vi "pco.camera_LightSheet_Example_IMAQ.vi"() -> ()   [LabVIEW 2019]
uses:
  pco.camera/Camera.lvclass
  pco.sdk/SpecialCommandsEdge/SpecialCommandsEdge.lvlib
panel:
  in  "dwExposureLines":u32=100
  in  "wTimeBase":u16(ring)=1 items=["ns", "us", "ms"]
  in  "dwLineTime":u32=50
  out "rawImage":u16[][](array[numeric])
  out "Image":T1(plugin-control)
  in  "data_format":T2(ring)=enum."Mono16"
  in  "Image Index":u32 max=99
  out "Recorded Images":u32
  in  "Quit":bool
  in  "roiY1":u64=2 min=2 max=1040 step=1
  in  "roiX1":u64=2 min=2 max=1392 step=1
  in  "roiY0":u64=1 min=1 max=1039 step=1
  in  "roiX0":u64=1 min=1 max=1391 step=1
  out "Image Height":u64
  out "Image Width":u64
  in  "dwImgCount":u32=10 caption="Required Number of Images" max=4023
  out "Error":errorcluster {"code" format="%x"}
  # "This example is similar to the simple example, but uses get/set line timeing for controlling the exposure.\nExposureTime = LineTime * ExposureLines\nBeside of the line timing part, a simple recording of an image sequence and the image access afterwards is done.\nIt is a good starting point for writing own applications, especially  for light sheet application development.\nBut it will not be fail save, i.e. doesnt react on errors, just handles them forward to the end\n\nUsage:\nSelect your required image count and the required line tiime + number of exposure lines before you start the program.\nOnce started, the camera class will be initialized and images will be recorded automatically.\nWhen acquisition has finished you can address the images and set a certain roi \nTo finish the program click on quit application, this will force fan exit of the camera class"
  # "pco.labview"
  # "Camera Setup"
  # "Recording Control"
  # "Parameters for image readout"
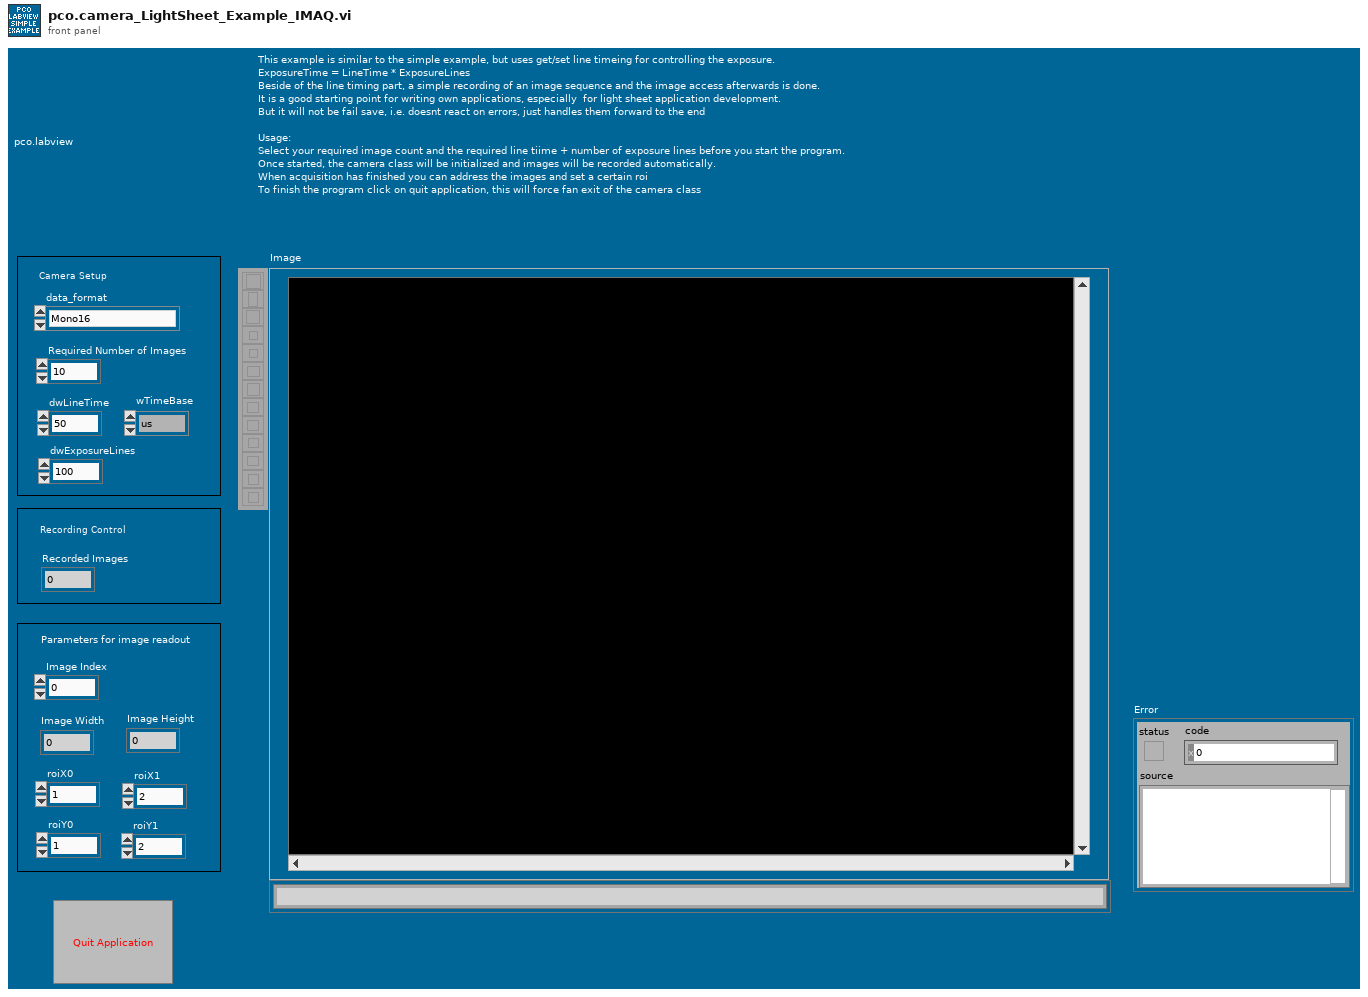
[diagram p1: front panel]
types:
  T1 = typedef "IMAQ Image.ctl" = refnum<image>
  T2 = enum16{"Undefined", "Mono8", "Mono16", "BGRA8", "RGBA8", "BGRA16", "RGBA16", "CompressedMono8"}
  T3 = enum8{"Enabled", "Disabled", "Disabled and Grayed Out"}
  T4 = enum16{"sequence", "sequence non blocking", "ring buffer", "fifo", "sequence_dpcore", "sequence_non_blocking_dpcore", "ring_buffer_dpcore", "fifo_dpcore", "tif", "multitif", "pcoraw", "b16", "dicom", "multidicom"}
  T5 = typedef "Image Type" = u32
  T6 = typedef "Camera.lvclass/binning.ctl" = cluster{"vert":u16, "horz":u16}
  T7 = cluster{"exposure_time_s":dbl, "delay_time_s":dbl, "roi":cluster{"x0":u64, "y0":u64, "x1":u64, "y1":u64}, "timestamp_mode":u16, "pixelrate":u32, "trigger_mode":u16, "acquire_mode":u16, "metadata_mode":u16, "noisefilter_mode":u16, "binning":T6}
  T8 = typedef "Color (U64)" = cluster{"Plane 3 (Blue)":u16, "Plane 2 (Green)":u16, "Plane 1 (Red)":u16, "Plane 4 (alpha)":u16}
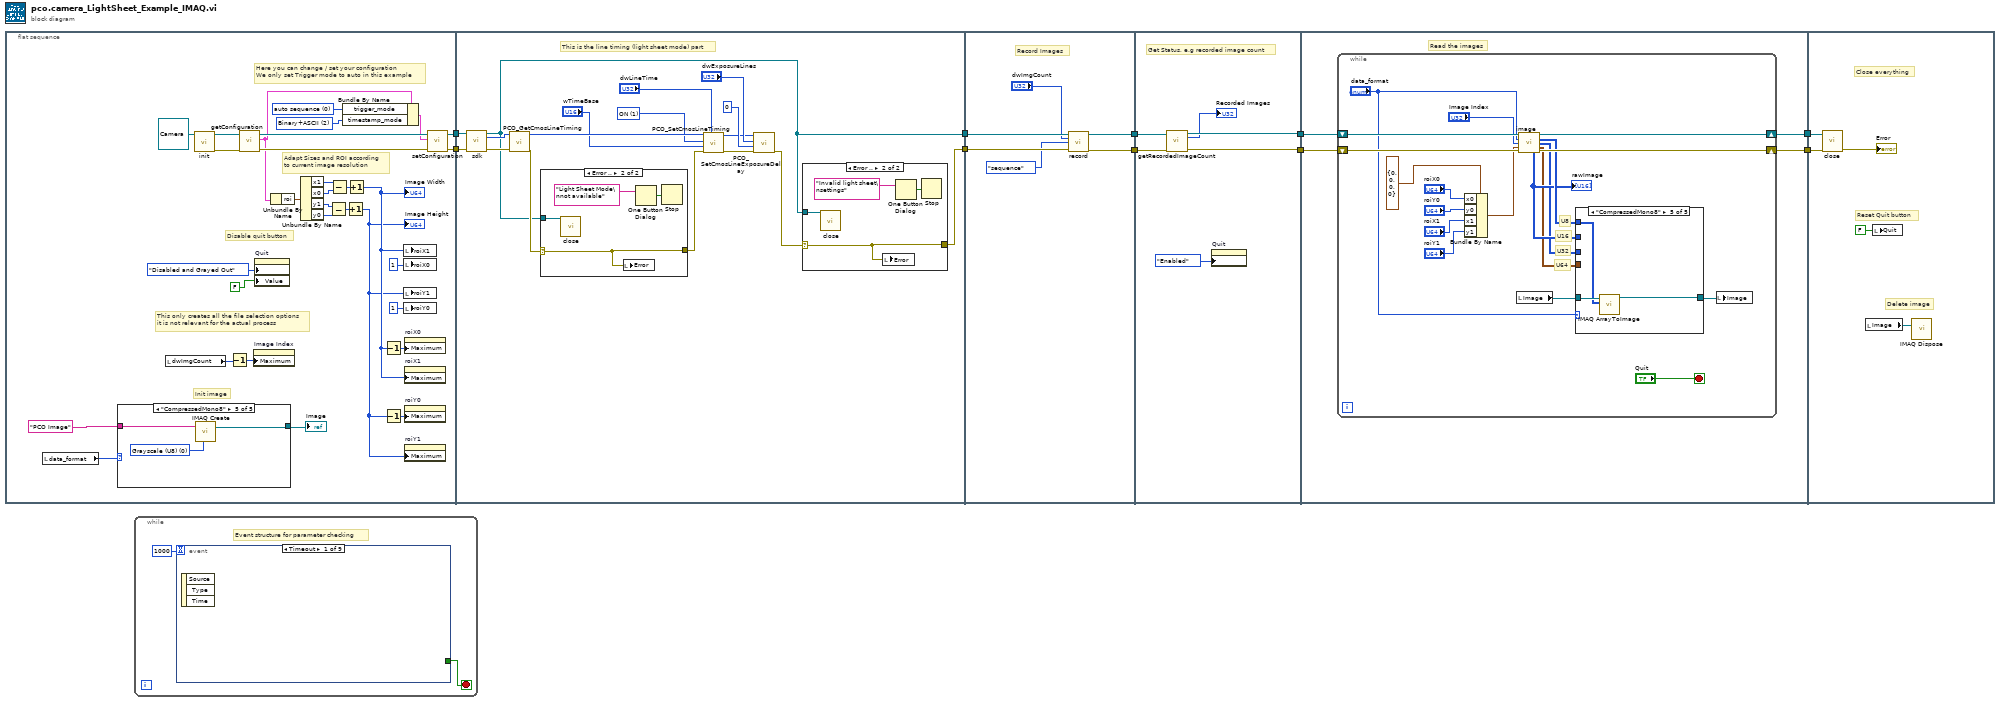
[diagram p0: block diagram]
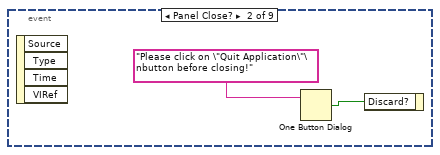
[diagram p2: hidden frame]
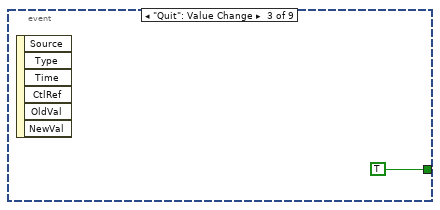
[diagram p3: hidden frame]
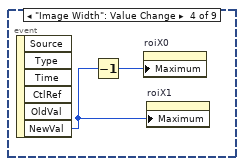
[diagram p4: hidden frame]
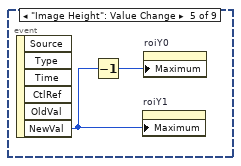
[diagram p5: hidden frame]
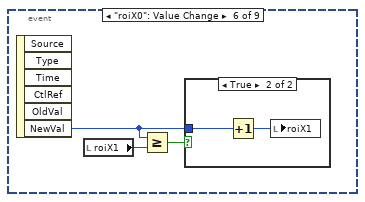
[diagram p6: hidden frame]
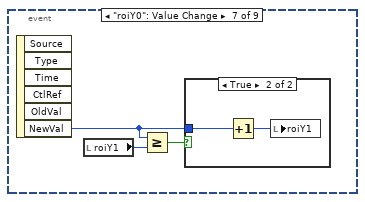
[diagram p8: hidden frame]
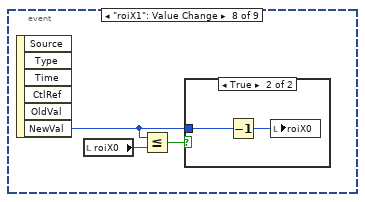
[diagram p10: hidden frame]
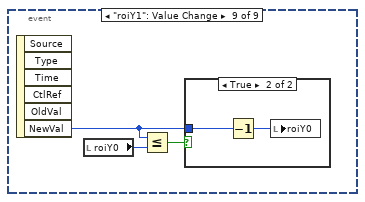
[diagram p12: hidden frame]
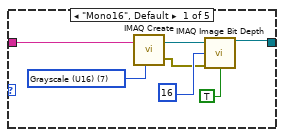
[diagram p14: hidden frame]
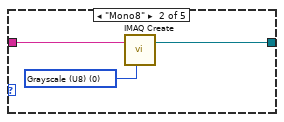
[diagram p15: hidden frame]
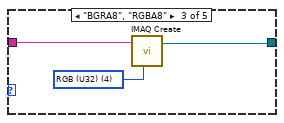
[diagram p16: hidden frame]
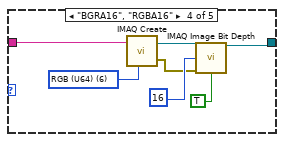
[diagram p17: hidden frame]
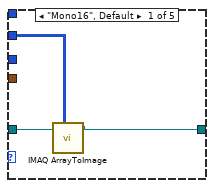
[diagram p20: hidden frame]
diagram:
  n1 = flat-sequence {
    tunnel: [w34] -> w4
    tunnel: [w33] -> w2
    tunnel: w4 -> [w77]
    tunnel: [w65] -> w3
    tunnel: w2 -> [w76]
    tunnel: [w66] -> w1
    tunnel: w3 -> [w97]
    tunnel: w1 -> [w96]
    tunnel: [w94] -> w10
    tunnel: [w93] -> w9
    tunnel: w10 -> [w103]
    tunnel: w9 -> [w102]
    tunnel: [w101] -> w8
    tunnel: [w100] -> w7
    tunnel: w8 -> [w106]
    tunnel: w7 -> [w107]
    tunnel: [w105] -> w6
    tunnel: [w104] -> w5
    tunnel: w6 -> [w144]
    tunnel: w5 -> [w143]
    frame #0 {
      w18 = u16 2 items=["OFF", "Binary", "Binary+ASCII", "ASCII"] ("TimestampMode")
      w38 = u16 0 items=["auto sequence"=0, "software trigger"=1, "external exposure start & software trigger"=2, "external exposure control"=3, "external synchronized"=4, "fast external exposure control"=5, "external CDS control"=6, "slow external exposure control"=7, "external synchronized HDSDI"=258] ("TriggerMode")
      # "Init image"
      # "This only creates all the file selection options\nit is not relevant for the actual process"
      # "Adapt Sizes and ROI according\nto current image resolution"
      # "Disable quit button"
      # "Here you can change / set your configuration\nWe only set Trigger mode to auto in this example"
      n2 = local read "data_format"() -> (w13:T2)
      n3 = case shown="\"CompressedMono8\"" w13 {
        tunnel: "PCO Image" ("Image Name") -> [w47 w51 w53 w60 w63]
        tunnel: [w42 w49 w52 w56 w62] -> w12
        frame "Mono16", Default {
          w48 = T5 7 items=["Grayscale (U8)", "Grayscale (I16)", "Grayscale (SGL)", "Complex (CSG)", "RGB (U32)", "HSL (U32)", "RGB (U64)", "Grayscale (U16)"] ("Image Type")
          n4 = call "IMAQ Create"("Image Name"=w47, "Image Type"=w48) -> ("New Image"=w44:T1, "error out"=w43:errorcluster)  [unwired: 3 in]
          n5 = call "IMAQ Image Bit Depth"("Image"=w44, "Bit Depth (0)"=u32 16, "error in (no error)"=w43, "Get/Set Bit Depth? (Set)"=TRUE) -> ("Image Out"=w42:T1)  [unwired: 9 in, 2 out]
        }
        frame "Mono8" {
          w50 = T5 0 items=["Grayscale (U8)", "Grayscale (I16)", "Grayscale (SGL)", "Complex (CSG)", "RGB (U32)", "HSL (U32)", "RGB (U64)", "Grayscale (U16)"] ("Image Type")
          n6 = call "IMAQ Create"("Image Name"=w51, "Image Type"=w50) -> ("New Image"=w49:T1)  [unwired: 3 in, 1 out]
        }
        frame "BGRA8", "RGBA8" {
          w54 = T5 4 items=["Grayscale (U8)", "Grayscale (I16)", "Grayscale (SGL)", "Complex (CSG)", "RGB (U32)", "HSL (U32)", "RGB (U64)", "Grayscale (U16)"] ("Image Type")
          n7 = call "IMAQ Create"("Image Name"=w53, "Image Type"=w54) -> ("New Image"=w52:T1)  [unwired: 3 in, 1 out]
        }
        frame "BGRA16", "RGBA16" {
          w61 = T5 6 items=["Grayscale (U8)", "Grayscale (I16)", "Grayscale (SGL)", "Complex (CSG)", "RGB (U32)", "HSL (U32)", "RGB (U64)", "Grayscale (U16)"] ("Image Type")
          n8 = call "IMAQ Create"("Image Name"=w60, "Image Type"=w61) -> ("New Image"=w57:T1, "error out"=w55:errorcluster)  [unwired: 3 in]
          n9 = call "IMAQ Image Bit Depth"("Image"=w57, "Bit Depth (0)"=u32 16, "error in (no error)"=w55, "Get/Set Bit Depth? (Set)"=TRUE) -> ("Image Out"=w56:T1)  [unwired: 9 in, 2 out]
        }
        frame "CompressedMono8" {
          w64 = T5 0 items=["Grayscale (U8)", "Grayscale (I16)", "Grayscale (SGL)", "Complex (CSG)", "RGB (U32)", "HSL (U32)", "RGB (U64)", "Grayscale (U16)"] ("Image Type")
          n10 = call "IMAQ Create"("Image Name"=w63, "Image Type"=w64) -> ("New Image"=w62:T1)  [unwired: 3 in, 1 out]
        }
      }
      "Image" <- w12
      n11 = local read "dwImgCount"() -> (w14:u32)
      n12 = call-dynamic "init.vi"("Camera in"=refnum<class "Camera.lvclass"> refnum ("PCOCamera in")) -> ("Camera out"=w40:refnum<class "Camera.lvclass">, "error out"=w39:errorcluster)  [unwired: 8 in]
      n13 = Decrement(x=w14) -> (x-1=w15:u32)
      n14 = call-dynamic "getConfiguration.vi"("error in (no error)"=w39, "Camera in"=w40) -> ("error out"=w36:errorcluster, "configuration"=w28:T7, "Camera out"=w37:refnum<class "Camera.lvclass">)  [unwired: 7 in]
      n15 = property on="Image Index" class="DigNum (strict)"("Maximum"=w15) -> ()  [unwired: 2 in, 2 out]
      n16 = property on="Quit" class="Bool (strict)"("DisabledEnum"=T3."Disabled and Grayed Out" ("Disabled"), "Value"=FALSE ("Stop")) -> ()  [unwired: 2 in, 2 out]
      n17 = Unbundle By Name(w28) -> ("roi"=w27:cluster{"x0":u64, "y0":u64, "x1":u64, "y1":u64})
      n18 = Unbundle By Name(w27) -> ("x1"=w25:u64, "x0"=w26:u64, "y1"=w23:u64, "y0"=w24:u64)
      n19 = Subtract(x=w23, y=w24) -> (x-y=w21:u64)
      n20 = Subtract(x=w25, y=w26) -> (x-y=w22:u64)
      n21 = Bundle By Name(cluster=w28, "trigger_mode"=w38, "timestamp_mode"=w18) -> (w35:T7)
      n22 = Increment(x=w21) -> (x+1=w19:u64)
      "Image Height" <- w19
      n23 = Increment(x=w22) -> (x+1=w20:u64)
      "Image Width" <- w20
      n24 = Decrement(x=w20) -> (x-1=w30:u64)
      n25 = Decrement(x=w19) -> (x-1=w29:u64)
      n26 = local write "roiX1"(w20) -> ()
      n27 = local write "roiX0"(u64 1 ("roiY0")) -> ()
      n28 = local write "roiY1"(w19) -> ()
      n29 = local write "roiY0"(u64 1 ("roiY0")) -> ()
      n30 = property on="roiX0" class="DigNum (strict)"("Maximum"=w30) -> ()  [unwired: 2 in, 2 out]
      n31 = property on="roiX1" class="DigNum (strict)"("Maximum"=w20) -> ()  [unwired: 2 in, 2 out]
      n32 = property on="roiY0" class="DigNum (strict)"("Maximum"=w29) -> ()  [unwired: 2 in, 2 out]
      n33 = property on="roiY1" class="DigNum (strict)"("Maximum"=w19) -> ()  [unwired: 2 in, 2 out]
      n34 = call-dynamic "setConfiguration.vi"("error in (no error)"=w36, "configuration"=w35, "Camera in"=w37) -> ("error out"=w33:errorcluster, "Camera out"=w34:refnum<class "Camera.lvclass">)  [unwired: 7 in]
    }
    frame #1 {
      w73 = u16 1 items=["OFF", "ON"] ("wParameter")
      # "This is the line timing (light sheet mode) part"
      n35 = call-dynamic "sdk.vi"("Camera in"=w77, "error in (no error)"=w76) -> ("Camera out"=w65:refnum<class "Camera.lvclass">, "sdk"=w75:u64, "error out"=w81:errorcluster)  [unwired: 11 in]
      n36 = call "PCO_GetCmosLineTiming.vi"("ph"=w75, "error in (no error)"=w81) -> ("ph out"=w74:u64, "error out"=w80:errorcluster)  [unwired: 10 in, 6 out]
      n37 = case shown="Error .." w80 {
        selector: w80 -> [w87 w88]
        tunnel: [w87 w88] -> w79
        tunnel: w65 -> [_ w89]
        frame No Error {
        }
        frame Error {
          n38 = call-dynamic "close.vi"("Camera in"=w89) -> ()  [unwired: 10 in, 1 out]
          n39 = local write "Error"(w88) -> ()
          n40 = One Button Dialog(message="Light Sheet Mode\nnot available") -> (true=w90:bool)  [unwired: 1 in]
          n41 = Stop(stop? (T)=w90) -> ()
        }
      }
      n42 = call "PCO_SetCmosLineTiming.vi"("dwLineTime"="dwLineTime", "error in (no error)"=w79, "wTimeBase"="wTimeBase", "wParameter"=w73, "ph"=w74) -> ("error out"=w78:errorcluster, "ph out"=w68:u64)  [unwired: 4 in, 1 out]
      n43 = call "PCO_SetCmosLineExposureDelay.vi"("error in (no error)"=w78, "dwDelayLines"=u32 0, "dwExposureLines"="dwExposureLines", "ph"=w68) -> ("error out"=w67:errorcluster)  [unwired: 5 in, 2 out]
      n44 = case shown="Error .." w67 {
        selector: w67 -> [w82 w83]
        tunnel: [w82 w83] -> w66
        tunnel: w65 -> [_ w84]
        frame No Error {
        }
        frame Error {
          n45 = call-dynamic "close.vi"("Camera in"=w84) -> ()  [unwired: 10 in, 1 out]
          n46 = local write "Error"(w83) -> ()
          n47 = One Button Dialog(message="Invalid light sheet\nsettings") -> (true=w85:bool)  [unwired: 1 in]
          n48 = Stop(stop? (T)=w85) -> ()
        }
      }
    }
    frame #2 {
      # "Record Images"
      n49 = call-dynamic "record.vi"("Camera in"=w97, "num_images"="dwImgCount", "record_mode"=T4."sequence", "error in (no error)"=w96) -> ("Camera out"=w94:refnum<class "Camera.lvclass">, "error out"=w93:errorcluster)  [unwired: 10 in]
    }
    frame #3 {
      # "Get Status, e.g recorded image count"
      n50 = call-dynamic "getRecordedImageCount.vi"("Camera in"=w103, "error in (no error)"=w102) -> ("Camera out"=w101:refnum<class "Camera.lvclass">, "recorded_image_count"=→"Recorded Images":u32, "error out"=w100:errorcluster)  [unwired: 11 in]
      n51 = property on="Quit" class="Bool (strict)"("DisabledEnum"=T3."Enabled" ("Disabled")) -> ()  [unwired: 2 in, 2 out]
    }
    frame #4 {
      # "Read the images"
      n52 = while {
        shift-right: [w124] -> w105
        shift-left: w106 -> [w126]
        shift-right: [w119] -> w104
        shift-left: w107 -> [w125]
        stop <- "Quit" stop-if-true
        # "U64"
        # "U32"
        # "U16"
        # "U8"
        n53 = Bundle By Name(cluster=cluster{"x0":u64, "y0":u64, "x1":u64, "y1":u64} {"x0"=0, "y0"=0, "x1"=0, "y1"=0} ("roi"), "x0"="roiX0", "y0"="roiY0", "x1"="roiX1", "y1"="roiY1") -> (w118:cluster{"x0":u64, "y0":u64, "x1":u64, "y1":u64})
        n54 = local read "Image"() -> (w111:T1)
        n55 = call-dynamic "image.vi"("Camera in"=w126, "data_format"="data_format", "image_index"="Image Index", "roi"=w118, "error in (no error)"=w125) -> ("Camera out"=w124:refnum<class "Camera.lvclass">, "image (U8)"=w115:u8[][], "image (U32)"=w113:u32[][], "image (U64)"=w112:T8[][], "raw_image (U16)"=w114:u16[][], "error out"=w119:errorcluster)  [unwired: 3 in, 2 out]
        "rawImage" <- w114
        n56 = case shown="\"CompressedMono8\"" "data_format" {
          tunnel: w111 -> [w129 w132 w135 w138 w141]
          tunnel: [w127 w130 w134 w136 w140] -> w110
          tunnel: w112 -> [_ _ _ w137 _]
          tunnel: w113 -> [_ _ w133 _ _]
          tunnel: w115 -> [_ w131 _ _ w139]
          tunnel: w114 -> [w128 _ _ _ _]
          frame "Mono16", Default {
            n57 = call "IMAQ ArrayToImage"("Image Pixels (U16)"=w128, "Image"=w129) -> ("Image Out"=w127:T1)  [unwired: 8 in, 1 out]
          }
          frame "Mono8" {
            n58 = call "IMAQ ArrayToImage"("Image Pixels (U8)"=w131, "Image"=w132) -> ("Image Out"=w130:T1)  [unwired: 8 in, 1 out]
          }
          frame "BGRA8", "RGBA8" {
            n59 = call "IMAQ ArrayToColorImage"("Image Pixels (U32)"=w133, "Image"=w135) -> ("Image Out"=w134:T1)  [unwired: 3 in, 1 out]
          }
          frame "BGRA16", "RGBA16" {
            n60 = call "IMAQ ArrayToColorImage"("Image"=w138, "Image Pixels (U64)"=w137) -> ("Image Out"=w136:T1)  [unwired: 3 in, 1 out]
          }
          frame "CompressedMono8" {
            n61 = call "IMAQ ArrayToImage"("Image Pixels (U8)"=w139, "Image"=w141) -> ("Image Out"=w140:T1)  [unwired: 8 in, 1 out]
          }
        }
        n62 = local write "Image"(w110) -> ()
      }
    }
    frame #5 {
      # "Delete image"
      # "Reset Quit button"
      # "Close everything"
      n63 = call-dynamic "close.vi"("error in (no error)"=w143, "Camera in"=w144) -> ("error out"=→"Error":errorcluster)  [unwired: 9 in]
      n64 = local read "Image"() -> (w142:T1)
      n65 = local write "Quit"(FALSE ("Stop")) -> ()
      n66 = call "IMAQ Dispose"("Image"=w142) -> ()  [unwired: 5 in, 1 out]
    }
  }
  n67 = while {
    stop <- w147 stop-if-true
    # "Event structure for parameter checking"
    n68 = event shown="[0] Timeout" {
      selector: _ -> [_ _ _ _ _ _ _ _ _]
      dyn-events: _ -> [_ _ _ _ _ _ _ _ _]
      timeout: 1000 -> [_ _ _ _ _ _ _ _ _]
      tunnel: [_ _ TRUE _ _ _ _ _ _] -> w147
      event Timeout {
        n69 = event-data() -> ()  [unwired: 1 in, 3 out]
      }
      event Panel Close? {
        n70 = event-data() -> ()  [unwired: 1 in, 4 out]
        n71 = One Button Dialog(message="Please click on \"Quit Application\"\nbutton before closing!") -> (true=w149:bool)  [unwired: 1 in]
        n72 = event-data("Discard?"=w149) -> ()  [unwired: 1 in, 1 out]
      }
      event "Quit": Value Change {
        n73 = event-data() -> ()  [unwired: 1 in, 6 out]
      }
      event "Image Width": Value Change {
        n74 = event-data() -> ("NewVal"=w152:u64)  [unwired: 1 in, 5 out]
        n75 = Decrement(x=w152) -> (x-1=w153:u64)
        n76 = property on="roiX0" class="DigNum (strict)"("Maximum"=w153) -> ()  [unwired: 2 in, 2 out]
        n77 = property on="roiX1" class="DigNum (strict)"("Maximum"=w152) -> ()  [unwired: 2 in, 2 out]
      }
      event "Image Height": Value Change {
        n78 = event-data() -> ("NewVal"=w154:u64)  [unwired: 1 in, 5 out]
        n79 = Decrement(x=w154) -> (x-1=w155:u64)
        n80 = property on="roiY1" class="DigNum (strict)"("Maximum"=w154) -> ()  [unwired: 2 in, 2 out]
        n81 = property on="roiY0" class="DigNum (strict)"("Maximum"=w155) -> ()  [unwired: 2 in, 2 out]
      }
      event "roiX0": Value Change {
        n82 = event-data() -> ("NewVal"=w156:u64)  [unwired: 1 in, 5 out]
        n83 = local read "roiX1"() -> (w158:u64)
        n84 = Greater Or Equal?(x=w156, y=w158) -> (x >= y?=w157:bool)
        n85 = case shown="True" w157 {
          tunnel: w156 -> [_ w160]
          frame False {
          }
          frame True {
            n86 = Increment(x=w160) -> (x+1=w159:u64)
            n87 = local write "roiX1"(w159) -> ()
          }
        }
      }
      event "roiY0": Value Change {
        n88 = event-data() -> ("NewVal"=w161:u64)  [unwired: 1 in, 5 out]
        n89 = local read "roiY1"() -> (w163:u64)
        n90 = Greater Or Equal?(x=w161, y=w163) -> (x >= y?=w162:bool)
        n91 = case shown="True" w162 {
          tunnel: w161 -> [_ w165]
          frame False {
          }
          frame True {
            n92 = Increment(x=w165) -> (x+1=w164:u64)
            n93 = local write "roiY1"(w164) -> ()
          }
        }
      }
      event "roiX1": Value Change {
        n94 = event-data() -> ("NewVal"=w166:u64)  [unwired: 1 in, 5 out]
        n95 = local read "roiX0"() -> (w168:u64)
        n96 = Less Or Equal?(x=w166, y=w168) -> (x <= y?=w167:bool)
        n97 = case shown="True" w167 {
          tunnel: w166 -> [_ w170]
          frame False {
          }
          frame True {
            n98 = Decrement(x=w170) -> (x-1=w169:u64)
            n99 = local write "roiX0"(w169) -> ()
          }
        }
      }
      event "roiY1": Value Change {
        n100 = event-data() -> ("NewVal"=w171:u64)  [unwired: 1 in, 5 out]
        n101 = local read "roiY0"() -> (w173:u64)
        n102 = Less Or Equal?(x=w171, y=w173) -> (x <= y?=w172:bool)
        n103 = case shown="True" w172 {
          tunnel: w171 -> [_ w175]
          frame False {
          }
          frame True {
            n104 = Decrement(x=w175) -> (x-1=w174:u64)
            n105 = local write "roiY0"(w174) -> ()
          }
        }
      }
    }
  }
